vi "Register Request.vi"(4 "Promise":refnum<class "Promise.lvclass">, 6 "Data Request":T1, 8 "error in (no error)":errorcluster, 10 "Needed Data":T3[](array[typedef]), 11 "Historian Module in":refnum<class "Historian Module.lvclass">) -> (0 "error out":errorcluster, 3 "Historian Module out":refnum<class "Historian Module.lvclass">)   [LabVIEW 2020, in "VolatusHistorian.lvlib" / "Historian Module.lvclass"]
uses:
  Historian Module.lvclass
  Needed Group Data.ctl
  Data Request.ctl
  Time Format.ctl
  lv-promises/Promises/Promise/Promise.lvclass
  Historian Module.lvclass/Historian Module.ctl
  VolatusHistorian.lvlib
  Pending Request.ctl
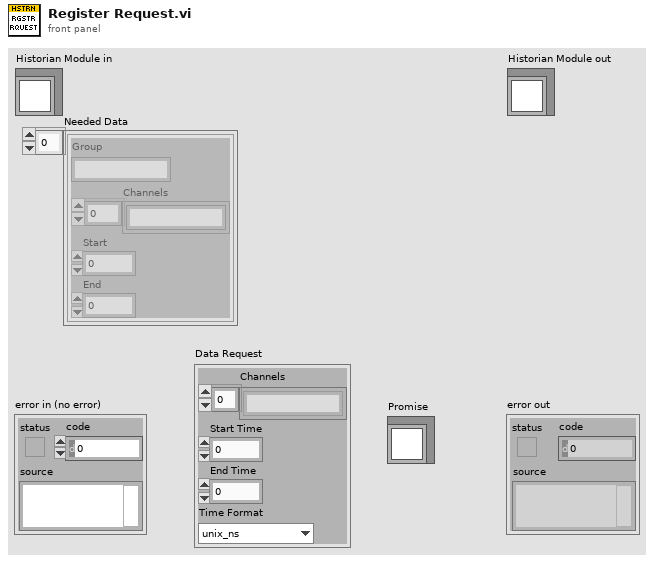
[diagram p1: front panel]
types:
  T1 = typedef "VolatusHistorian.lvlib/Data Request.ctl" = cluster{"Channels":string[], "Start Time":dbl, "End Time":dbl, "Time Format":T2}
  T2 = typedef "VolatusHistorian.lvlib/Time Format.ctl" = enum16{"unix_ns", "lv"}
  T3 = typedef "VolatusHistorian.lvlib/Historian Module.lvclass/Needed Group Data.ctl" = cluster{"Group":string, "Channels":string[], "Start":dbl, "End":dbl}
  T4 = typedef "VolatusHistorian.lvlib/Historian Module.lvclass/Pending Request.ctl" = cluster{"Request":T1, "Promise":refnum<class "Promise.lvclass">, "Pending Data":T3[]}
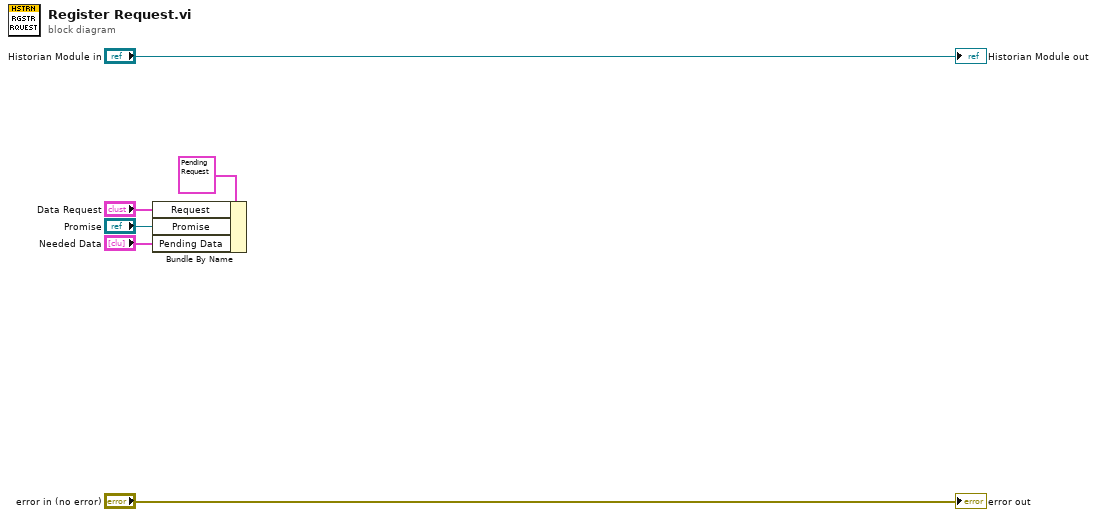
[diagram p0: block diagram]
diagram:
  n1 = Bundle By Name(cluster=T4 {"Request"={"Channels"=[], "Start Time"=0.0, "End Time"=0.0, "Time Format"=enum."unix_ns"}, "Promise"=refnum, "Pending Data"=[]} ("Pending Request"), "Request"="Data Request", "Promise"="Promise", "Pending Data"="Needed Data") -> ()  [unwired: 1 out]
  "error out" <- "error in (no error)"
  "Historian Module out" <- "Historian Module in"
